vi "Read Test Case object from front panel control.vi"(8 "error in (no error)":errorcluster, 11 "LUnit Test Case In":refnum<class "LUnit Test Case.lvclass">) -> (0 "error out":errorcluster, 3 "LUnit Test Case Out":refnum<class "LUnit Test Case.lvclass">)   [LabVIEW 2020, in "LUnit Test Case.lvclass"]
uses:
  LUnit Test Case.lvclass
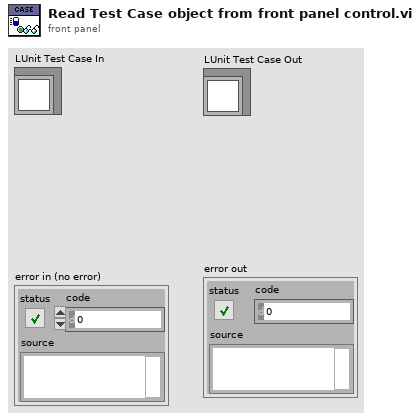
[diagram p1: front panel]
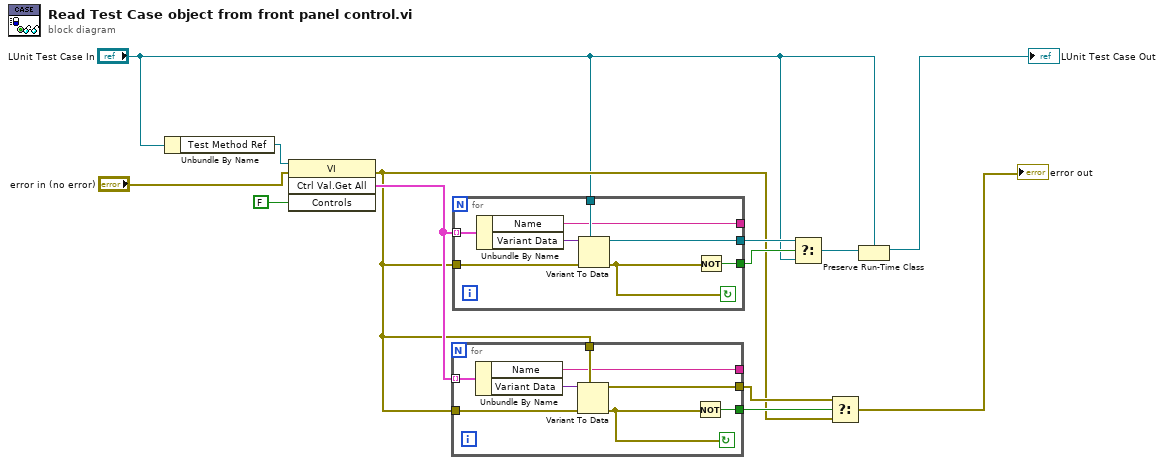
[diagram p0: block diagram]
diagram:
  n1 = Unbundle By Name("LUnit Test Case In") -> ("Test Method Ref"=w8:refnum<vi>)
  n2 = invoke on="Invoke Node" class="VI" method="Ctrl Val.Get All"(reference=w8, error in="error in (no error)", "Controls"=FALSE) -> (error out=w4:errorcluster, "Get All Control Values Variant"=w7:cluster{"Name":string, "Variant Data":variant}[])  [unwired: 1 in, 2 out]
  n3 = for {
    tunnel: w7 -> [w21] mode=indexing
    tunnel: w4 -> [w19]
    tunnel: [w18] -> _
    tunnel: [w14] -> w6
    tunnel: [w16] -> w5
    tunnel: w4 -> [w15]
    stop <- w17 continue-if-true
    n4 = Unbundle By Name(w21) -> ("Name"=w18:string, "Variant Data"=w20:variant)
    n5 = Variant To Data(error in=w15, type=w19, Variant=w20) -> (data=w16:errorcluster, error out=w17:errorcluster)
    n6 = Not(x=w17) -> (.not. x?=w14:bool)
  }
  n7 = for {
    tunnel: w7 -> [w29] mode=indexing
    tunnel: "LUnit Test Case In" -> [w27]
    tunnel: [w26] -> _
    tunnel: [w22] -> w10
    tunnel: [w24] -> w9
    tunnel: w4 -> [w23]
    stop <- w25 continue-if-true
    n8 = Unbundle By Name(w29) -> ("Name"=w26:string, "Variant Data"=w28:variant)
    n9 = Variant To Data(error in=w23, type=w27, Variant=w28) -> (data=w24:refnum<class "LUnit Test Case.lvclass">, error out=w25:errorcluster)
    n10 = Not(x=w25) -> (.not. x?=w22:bool)
  }
  n11 = Select(t=w9, s=w10, f="LUnit Test Case In") -> (s? t:f=w12:refnum<class "LUnit Test Case.lvclass">)
  n12 = Select(t=w5, s=w6, f=w4) -> (s? t:f=→"error out":errorcluster)
  n13 = Preserve Run-Time Class(object in=w12, 2:"LUnit Test Case In") -> (object out=→"LUnit Test Case Out":refnum<class "LUnit Test Case.lvclass">)  [unwired: 1 in, 1 out]
